vi "Elevator.vi"(8 "actuating axis":dbl, 11 "Elevator Locked?":bool) -> (0 "Winch Setpoint":dbl)   [LabVIEW 2014]
uses:
  <vilib>/Rock Robotics/Network Tables/SD Read Boolean.vi
  Robot Global Data.vi
panel:
  out "Winch Motor speed 2":dbl
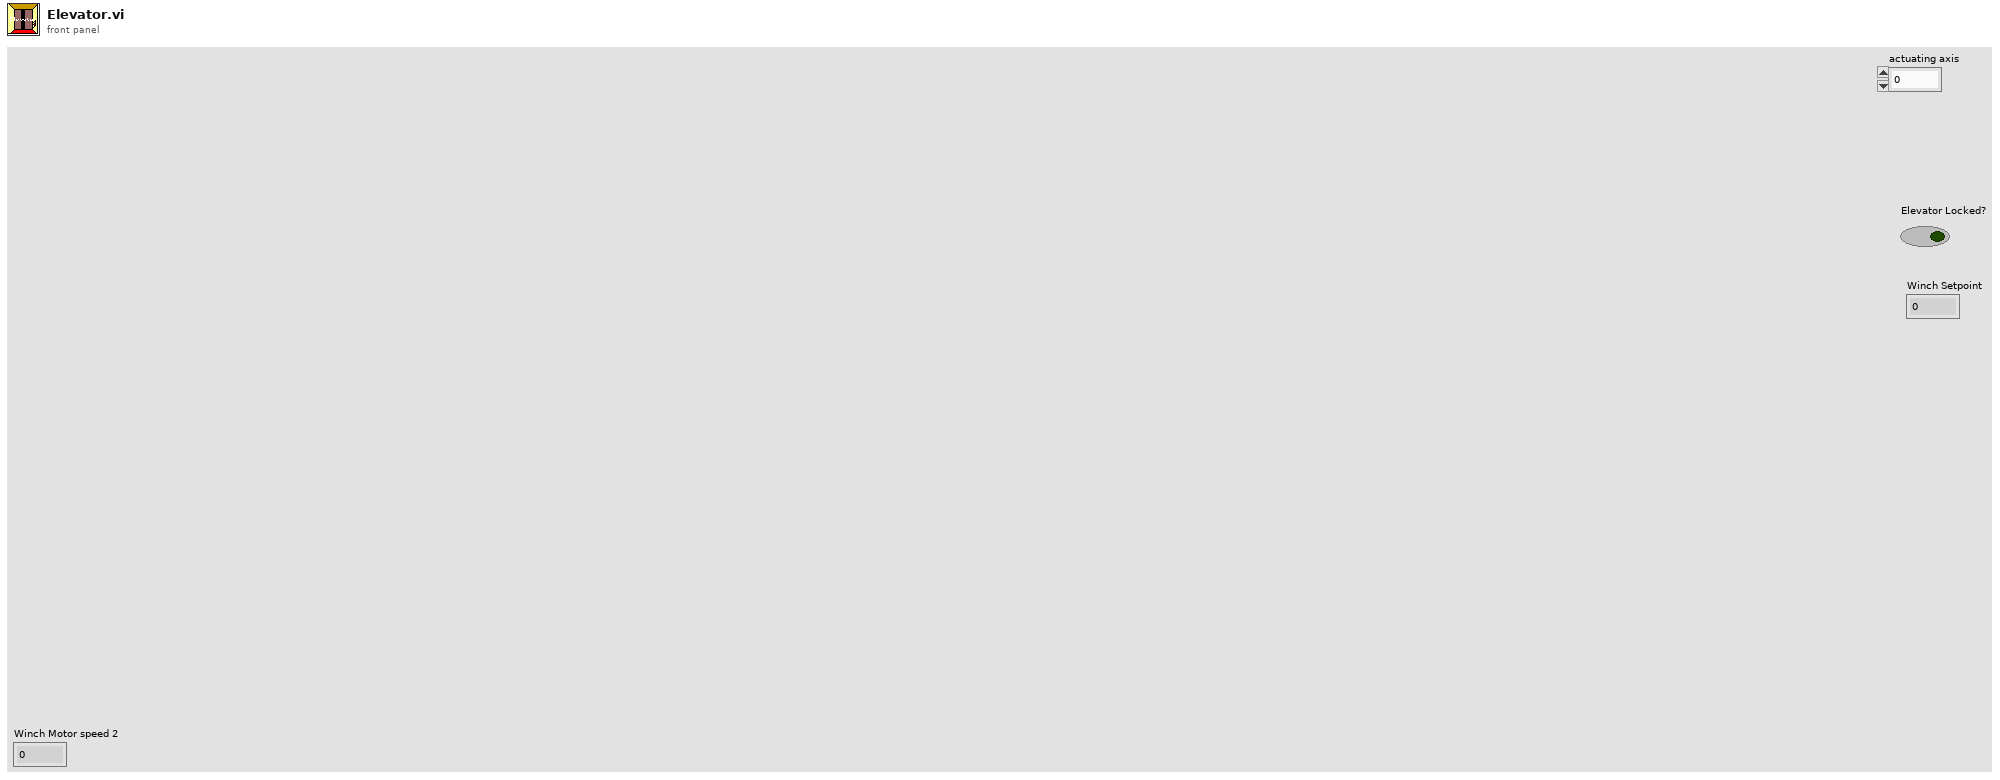
[diagram p1: front panel]
types:
  T1 = typedef "WPI_DigitalInputDevRef.ctl" = cluster{"DevStatus":errorcluster, "DIO Channel":T2, "Controller":T3}
  T2 = typedef "FPGA_DIOChannel.ctl" = enum8{"DIO 0", "DIO 1", "DIO 2", "DIO 3", "DIO 4", "DIO 5", "DIO 6", "DIO 7", "DIO 8", "DIO 9", "DIO MXP 0", "DIO MXP 1", "DIO MXP 2", "DIO MXP 3", "DIO MXP 4", "DIO MXP 5", "DIO MXP 6", "DIO MXP 7", "DIO MXP 8", "DIO MXP 9", "DIO MXP 10", "DIO MXP 11", "DIO MXP 12", "DIO MXP 13", "DIO MXP 14", "DIO MXP 15", "Invalid"}
  T3 = typedef "FPGA_TypedefDigitalModule.ctl" = enum16{"Controller 1"}
  T4 = typedef "WPI_MotorControlDeviceRef.ctl" = cluster{"DeviceStatus":errorcluster, "Type":T5, "PWM":cluster{"Controller":T3, "PWM Channel":T6, "DeadBand":T7}, "CAN":cluster{"Device Number":u8, "Control Mode":T8, "Semaphore":T9, "Max Vout":dbl, "TalonSRX Control Mode":T10}, "Invert":bool, "TransformRef":T11, "InvTransformRef":T11}
  T5 = typedef "WPI_MotorControlType.ctl" = enum16{"PWM", "CAN", "CANTalonSRX"}
  T6 = typedef "FPGA_DIOPWMChannel.ctl" = enum8{"PWM 0", "PWM 1", "PWM 2", "PWM 3", "PWM 4", "PWM 5", "PWM 6", "PWM 7", "PWM 8", "PWM 9", "PWM MXP 0", "PWM MXP 1", "PWM MXP 2", "PWM MXP 3", "PWM MXP 4", "PWM MXP 5", "PWM MXP 6", "PWM MXP 7", "PWM MXP 8", "PWM MXP 9", "Invalid"}
  T7 = typedef "WPI_PWMDeadband.ctl" = cluster{"Name":string, "maxPositivePwm":i32, "minPositivePwm":i32, "centerPwm":i32, "maxNegativePwm":i32, "minNegativePwm":i32, "angularRange":u16}
  T8 = typedef "WPI_CANJaguar_ControlMode.ctl" = enum8{"Percent VBus", "Current", "Speed", "Position", "Voltage"}
  T9 = typedef "Semaphore RefNum" = refnum<k1>
  T10 = typedef "WPI_CANTalonSRX_APIControlMode.ctl" = enum8{"Percent VBus", "Speed", "Position", "Slave", "Unchanged / Invalid"}
  T11 = typedef "WPI_PWMTransform_ConPane.ctl" = refnum<vi>
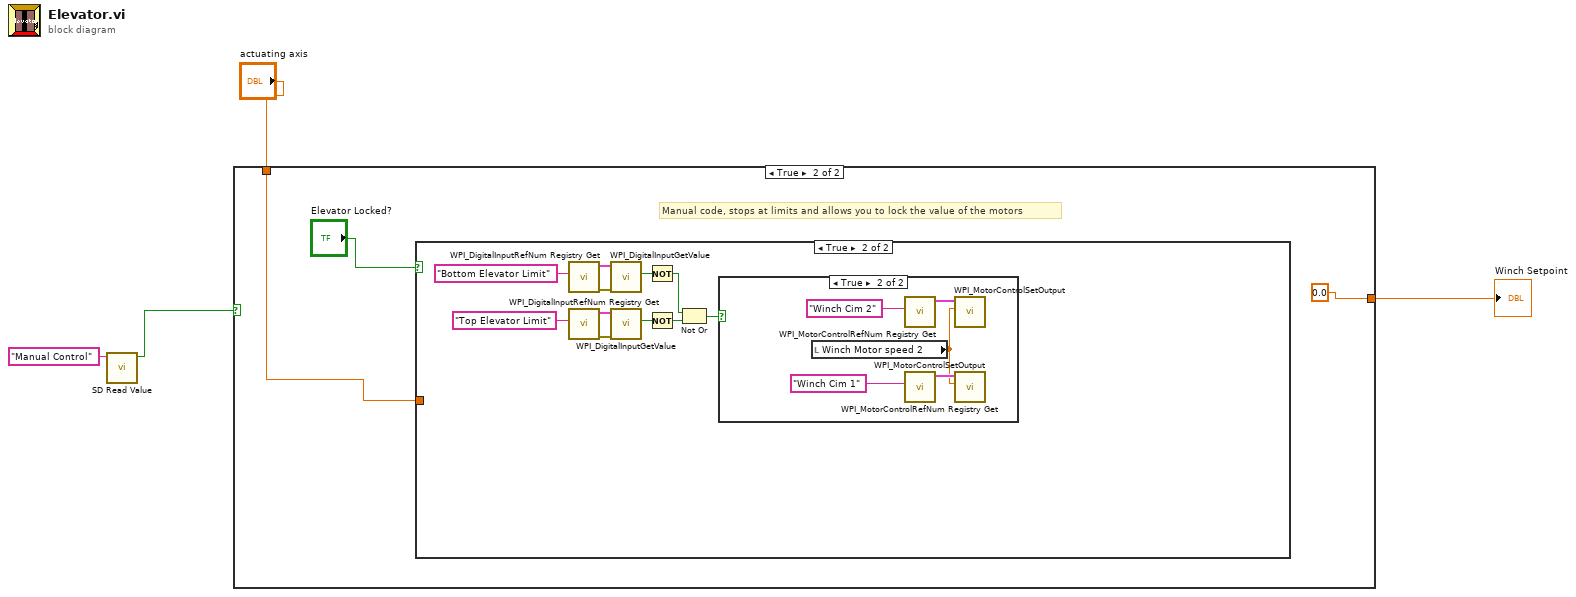
[diagram p0: block diagram]
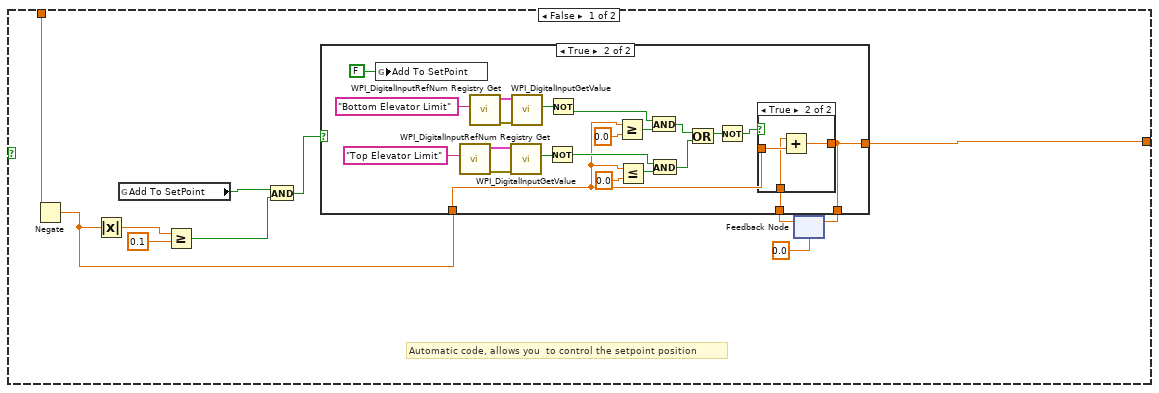
[diagram p2: hidden frame]
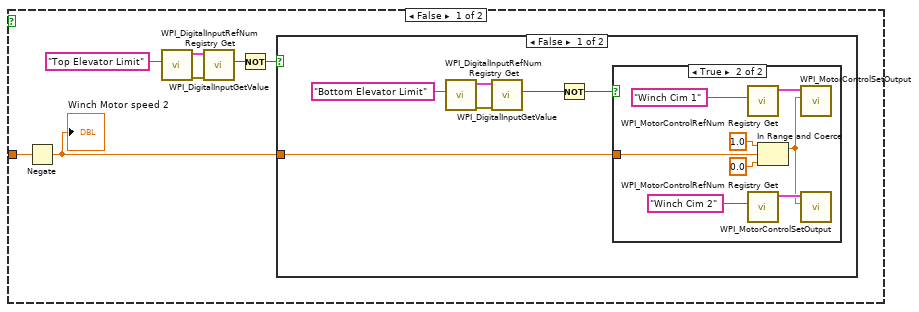
[diagram p5: hidden frame]
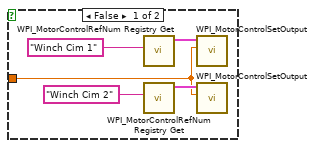
[diagram p6: hidden frame]
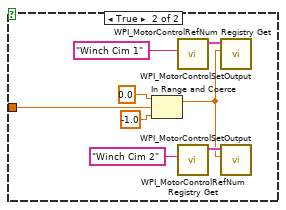
[diagram p7: hidden frame]
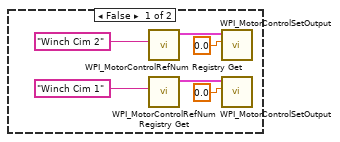
[diagram p8: hidden frame]
diagram:
  n1 = call-poly <vilib>:"SD Read Value.vi"("Name"="Manual Control") -> ("Boolean"=w1:bool)  [unwired: 8 in, 2 out]
  n2 = case shown="True" w1 {
    tunnel: "actuating axis" -> [w15 w43]
    tunnel: [w8 0.0] -> w3
    frame False {
      # "Automatic code, allows you  to control the setpoint position"
      n3 = Negate(x=w15) -> (-x=w9:dbl)
      n4 = Absolute Value(x=w9) -> (abs(x)=w13:dbl)
      n5 = global read "Robot Global Data.vi" "Add To SetPoint"() -> (w10:bool)
      n6 = Greater Or Equal?(x=w13, y=0.1) -> (x >= y?=w11:bool)
      n7 = And(x=w10, y=w11) -> (x .and. y?=w12:bool)
      n8 = feedback #1(0.0) -> (w5:dbl)
      n9 = case shown="True" w12 {
        tunnel: w9 -> [_ w21]
        tunnel: [w16 w20] -> w8
        tunnel: [w16 w20] -> w6
        tunnel: w5 -> [w16 w19]
        frame False {
        }
        frame True {
          n10 = global write "Robot Global Data.vi" "Add To SetPoint"(FALSE) -> ()
          n11 = call <vilib>:"WPI_DigitalInputRefNum Registry Get.vi"("refnum name"="Top Elevator Limit") -> ("error out"=w32:errorcluster, "DigitalInputDevRef"=w33:T1)  [unwired: 9 in]
          n12 = call <vilib>:"WPI_DigitalInputRefNum Registry Get.vi"("refnum name"="Bottom Elevator Limit") -> ("error out"=w37:errorcluster, "DigitalInputDevRef"=w36:T1)  [unwired: 9 in]
          n13 = call <vilib>:"WPI_DigitalInputGetValue.vi"("error in (no error)"=w32, "DigitalInputDevRef"=w33) -> ("Value"=w30:bool)  [unwired: 7 in, 2 out]
          n14 = call <vilib>:"WPI_DigitalInputGetValue.vi"("error in (no error)"=w37, "DigitalInputDevRef"=w36) -> ("Value"=w35:bool)  [unwired: 7 in, 2 out]
          n15 = Not(x=w30) -> (.not. x?=w28:bool)
          n16 = Not(x=w35) -> (.not. x?=w24:bool)
          n17 = Greater Or Equal?(x=w21, y=0.0) -> (x >= y?=w25:bool)
          n18 = Less Or Equal?(x=w21, y=0.0) -> (x <= y?=w27:bool)
          n19 = And(x=w24, y=w25) -> (x .and. y?=w23:bool)
          n20 = And(x=w28, y=w27) -> (x .and. y?=w22:bool)
          n21 = Or(x=w23, y=w22) -> (x .or. y?=w17:bool)
          n22 = Not(x=w17) -> (.not. x?=w18:bool)
          n23 = case shown="True" w18 {
            tunnel: [w39 w42] -> w20
            tunnel: w21 -> [_ w41]
            tunnel: w19 -> [w39 w40]
            frame False {
            }
            frame True {
              n24 = Add(x=w40, y=w41) -> (x+y=w42:dbl)
            }
          }
        }
      }
      n25 = feedback-in #1(w6) -> ()
    }
    frame True {
      # "Manual code, stops at limits and allows you to lock the value of the motors"
      n26 = case shown="True" "Elevator Locked?" {
        tunnel: w43 -> [w51 _]
        frame False {
          n27 = Negate(x=w51) -> (-x=w46:dbl)
          "Winch Motor speed 2" <- w46
          n28 = call <vilib>:"WPI_DigitalInputRefNum Registry Get.vi"("refnum name"="Top Elevator Limit") -> ("error out"=w49:errorcluster, "DigitalInputDevRef"=w50:T1)  [unwired: 9 in]
          n29 = call <vilib>:"WPI_DigitalInputGetValue.vi"("error in (no error)"=w49, "DigitalInputDevRef"=w50) -> ("Value"=w47:bool)  [unwired: 7 in, 2 out]
          n30 = Not(x=w47) -> (.not. x?=w52:bool)
          n31 = case shown="False" w52 {
            tunnel: w46 -> [w57 w74]
            frame False {
              n32 = call <vilib>:"WPI_DigitalInputRefNum Registry Get.vi"("refnum name"="Bottom Elevator Limit") -> ("error out"=w56:errorcluster, "DigitalInputDevRef"=w55:T1)  [unwired: 9 in]
              n33 = call <vilib>:"WPI_DigitalInputGetValue.vi"("error in (no error)"=w56, "DigitalInputDevRef"=w55) -> ("Value"=w53:bool)  [unwired: 7 in, 2 out]
              n34 = Not(x=w53) -> (.not. x?=w58:bool)
              n35 = case shown="True" w58 {
                tunnel: w57 -> [w59 w66]
                frame False {
                  n36 = call <vilib>:"WPI_MotorControlRefNum Registry Get.vi"("refnum name"="Winch Cim 1") -> ("MotorControlDevRef"=w61:T4)  [unwired: 9 in, 1 out]
                  n37 = call <vilib>:"WPI_MotorControlRefNum Registry Get.vi"("refnum name"="Winch Cim 2" ("Name")) -> ("MotorControlDevRef"=w62:T4)  [unwired: 9 in, 1 out]
                  n38 = call <vilib>:"WPI_MotorControlSetOutput.vi"("Output"=w59, "MotorControlDevRef"=w61) -> ()  [unwired: 7 in, 3 out]
                  n39 = call <vilib>:"WPI_MotorControlSetOutput.vi"("Output"=w59, "MotorControlDevRef"=w62) -> ()  [unwired: 7 in, 3 out]
                }
                frame True {
                  n40 = call <vilib>:"WPI_MotorControlRefNum Registry Get.vi"("refnum name"="Winch Cim 1") -> ("MotorControlDevRef"=w67:T4)  [unwired: 9 in, 1 out]
                  n41 = call <vilib>:"WPI_MotorControlRefNum Registry Get.vi"("refnum name"="Winch Cim 2" ("Name")) -> ("MotorControlDevRef"=w68:T4)  [unwired: 9 in, 1 out]
                  n42 = In Range and Coerce(upper limit=1.0, x=w66, lower limit=0.0) -> (coerced(x)=w64:dbl)  [unwired: 1 out]
                  n43 = call <vilib>:"WPI_MotorControlSetOutput.vi"("Output"=w64, "MotorControlDevRef"=w67) -> ()  [unwired: 7 in, 3 out]
                  n44 = call <vilib>:"WPI_MotorControlSetOutput.vi"("Output"=w64, "MotorControlDevRef"=w68) -> ()  [unwired: 7 in, 3 out]
                }
              }
            }
            frame True {
              n45 = In Range and Coerce(upper limit=0.0, x=w74, lower limit=-1.0) -> (coerced(x)=w72:dbl)  [unwired: 1 out]
              n46 = call <vilib>:"WPI_MotorControlRefNum Registry Get.vi"("refnum name"="Winch Cim 1") -> ("MotorControlDevRef"=w75:T4)  [unwired: 9 in, 1 out]
              n47 = call <vilib>:"WPI_MotorControlRefNum Registry Get.vi"("refnum name"="Winch Cim 2" ("Name")) -> ("MotorControlDevRef"=w76:T4)  [unwired: 9 in, 1 out]
              n48 = call <vilib>:"WPI_MotorControlSetOutput.vi"("Output"=w72, "MotorControlDevRef"=w75) -> ()  [unwired: 7 in, 3 out]
              n49 = call <vilib>:"WPI_MotorControlSetOutput.vi"("Output"=w72, "MotorControlDevRef"=w76) -> ()  [unwired: 7 in, 3 out]
            }
          }
        }
        frame True {
          n50 = call <vilib>:"WPI_DigitalInputRefNum Registry Get.vi"("refnum name"="Bottom Elevator Limit") -> ("error out"=w90:errorcluster, "DigitalInputDevRef"=w89:T1)  [unwired: 9 in]
          n51 = call <vilib>:"WPI_DigitalInputRefNum Registry Get.vi"("refnum name"="Top Elevator Limit") -> ("error out"=w85:errorcluster, "DigitalInputDevRef"=w86:T1)  [unwired: 9 in]
          n52 = call <vilib>:"WPI_DigitalInputGetValue.vi"("error in (no error)"=w90, "DigitalInputDevRef"=w89) -> ("Value"=w88:bool)  [unwired: 7 in, 2 out]
          n53 = call <vilib>:"WPI_DigitalInputGetValue.vi"("error in (no error)"=w85, "DigitalInputDevRef"=w86) -> ("Value"=w84:bool)  [unwired: 7 in, 2 out]
          n54 = Not(x=w88) -> (.not. x?=w82:bool)
          n55 = Not(x=w84) -> (.not. x?=w81:bool)
          n56 = Not Or(1:w81, 2:w82) -> (0:w80:bool)
          n57 = case shown="True" w80 {
            frame False {
              n58 = call <vilib>:"WPI_MotorControlRefNum Registry Get.vi"("refnum name"="Winch Cim 2") -> ("MotorControlDevRef"=w93:T4)  [unwired: 9 in, 1 out]
              n59 = call <vilib>:"WPI_MotorControlRefNum Registry Get.vi"("refnum name"="Winch Cim 1") -> ("MotorControlDevRef"=w96:T4)  [unwired: 9 in, 1 out]
              n60 = call <vilib>:"WPI_MotorControlSetOutput.vi"("Output"=0.0, "MotorControlDevRef"=w93) -> ()  [unwired: 7 in, 3 out]
              n61 = call <vilib>:"WPI_MotorControlSetOutput.vi"("Output"=0.0, "MotorControlDevRef"=w96) -> ()  [unwired: 7 in, 3 out]
            }
            frame True {
              n62 = local read "Winch Motor speed 2"() -> (w97:dbl)
              n63 = call <vilib>:"WPI_MotorControlRefNum Registry Get.vi"("refnum name"="Winch Cim 2" ("Name")) -> ("MotorControlDevRef"=w100:T4)  [unwired: 9 in, 1 out]
              n64 = call <vilib>:"WPI_MotorControlRefNum Registry Get.vi"("refnum name"="Winch Cim 1") -> ("MotorControlDevRef"=w99:T4)  [unwired: 9 in, 1 out]
              n65 = call <vilib>:"WPI_MotorControlSetOutput.vi"("Output"=w97, "MotorControlDevRef"=w100) -> ()  [unwired: 7 in, 3 out]
              n66 = call <vilib>:"WPI_MotorControlSetOutput.vi"("Output"=w97, "MotorControlDevRef"=w99) -> ()  [unwired: 7 in, 3 out]
            }
          }
        }
      }
    }
  }
  "Winch Setpoint" <- w3
